vi "Low Update.vi"(8 "error in":errorcluster, 10 "Input High":string, 11 "SerDes in":refnum<class "OOPbyRef.lvclass">) -> (0 "error out":errorcluster, 3 "SerDes out":refnum<class "OOPbyRef.lvclass">)   [LabVIEW 2021, in "DQMH_byOOPRef.lvlib" / "OOPbyRef.lvclass"]
uses:
  OOPbyRef.lvclass
  OOPbyRef.lvclass/OOPbyRef.ctl
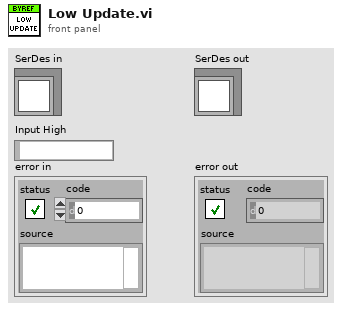
[diagram p1: front panel]
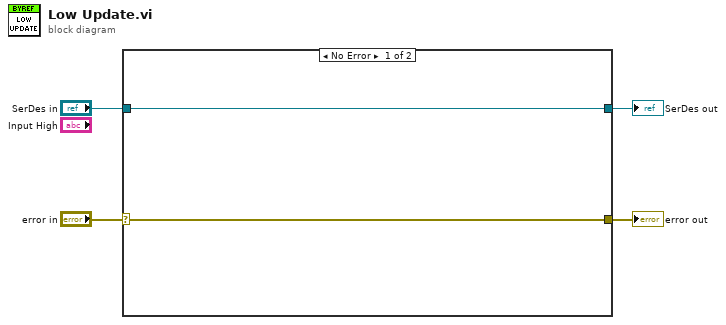
[diagram p0: block diagram]
diagram:
  n1 = case shown="No Error" "error in" {
    selector: "error in" -> [w6 w8]
    tunnel: [w6 w8] -> w3
    tunnel: [w5 w7] -> w1
    tunnel: "SerDes in" -> [w5 w7]
    frame No Error {
    }
    frame Error {
    }
  }
  "error out" <- w3
  "SerDes out" <- w1
